vi "Test Write Enums.vi"(11 "TwinCAT ADS in":refnum<class "TwinCAT ADS.lvclass">) -> (3 "TwinCAT ADS out":refnum<class "TwinCAT ADS.lvclass">)   [LabVIEW 2018]
uses:
  TwinCAT ADS Class/TwinCAT ADS.lvclass
  Controls/Enum.ctl
  67abcce4-d906-4956-a77e-4a47c9dde040.vi
  c0c5b84e-43cd-4ba1-b01f-cca28dc7bea8.vi
  903064a7-6281-4536-8159-57f8726da337.vi
  a8d287bd-4485-4814-8cd1-9655769c98e5.vi
  TwinCAT ADS Class/VIs/Data/Read.vi
  <vilib>/addons/_JKI Toolkits/Caraya/classes/Assert/Assert Equal Value_Variant.vi
  <vilib>/addons/_JKI Toolkits/Caraya/classes/Test/Test.lvclass
  <vilib>/addons/_JKI Toolkits/Caraya/classes/Assert/Assert.lvclass
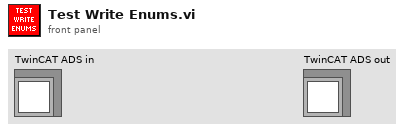
[diagram p1: front panel]
types:
  T1 = typedef "Enum.ctl" = enum16{"Member 0", "Member 1", "Member 2"}
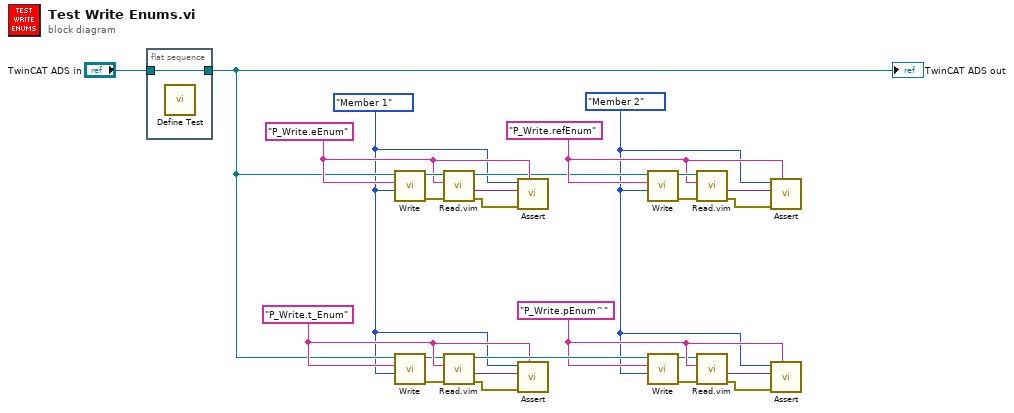
[diagram p0: block diagram]
diagram:
  w1 = Enum."Member 2" ("Enum")
  w2 = Enum."Member 1" ("Enum")
  w13 = "P_Write.pEnum^" ("Symbol Name")
  w8 = "P_Write.t_Enum" ("Symbol Name")
  w16 = "P_Write.refEnum" ("Symbol Name")
  w21 = "P_Write.eEnum" ("Symbol Name")
  n1 = flat-sequence {
    tunnel: "TwinCAT ADS in" -> [w27]
    tunnel: [w27] -> w3
    frame #0 {
      n2 = call <vilib>:"Define Test.vi"() -> ()  [unwired: 10 in, 2 out]
    }
  }
  n3 = call "Write.vi"("Value"=w2, "Symbol Name"=w21, "TwinCAT ADS in"=w3) -> ("error out"=w24:errorcluster, "TwinCAT ADS out"=w25:refnum<class "TwinCAT ADS.lvclass">)  [unwired: 7 in]
  n4 = call "Write.vi"("Value"=w2, "Symbol Name"=w8, "TwinCAT ADS in"=w3) -> ("error out"=w5:errorcluster, "TwinCAT ADS out"=w4:refnum<class "TwinCAT ADS.lvclass">)  [unwired: 7 in]
  n5 = call "Read.vim"("error in (no error)"=w24, "Symbol Name"=w21, "TwinCAT ADS in"=w25) -> ("error out"=w23:errorcluster, "Value"=w22:variant, "TwinCAT ADS out"=w15:refnum<class "TwinCAT ADS.lvclass">)  [unwired: 6 in]
  n6 = call "Read.vim"("error in (no error)"=w5, "Symbol Name"=w8, "TwinCAT ADS in"=w4) -> ("error out"=w6:errorcluster, "Value"=w7:variant, "TwinCAT ADS out"=w14:refnum<class "TwinCAT ADS.lvclass">)  [unwired: 6 in]
  n7 = call-poly <vilib>:"Assert.vi"("Label"=w21, "error in (no error)"=w23, "Y"=w22, "X"=w2) -> ()  [unwired: 6 in, 2 out]
  n8 = call-poly <vilib>:"Assert.vi"("Label"=w8, "error in (no error)"=w6, "Y"=w7, "X"=w2) -> ()  [unwired: 6 in, 2 out]
  n9 = call "Write.vi"("Value"=w1, "Symbol Name"=w16, "TwinCAT ADS in"=w15) -> ("error out"=w19:errorcluster, "TwinCAT ADS out"=w20:refnum<class "TwinCAT ADS.lvclass">)  [unwired: 7 in]
  n10 = call "Write.vi"("Value"=w1, "Symbol Name"=w13, "TwinCAT ADS in"=w14) -> ("error out"=w10:errorcluster, "TwinCAT ADS out"=w9:refnum<class "TwinCAT ADS.lvclass">)  [unwired: 7 in]
  n11 = call "Read.vim"("error in (no error)"=w19, "Symbol Name"=w16, "TwinCAT ADS in"=w20) -> ("error out"=w18:errorcluster, "Value"=w17:variant)  [unwired: 6 in, 1 out]
  n12 = call "Read.vim"("error in (no error)"=w10, "Symbol Name"=w13, "TwinCAT ADS in"=w9) -> ("error out"=w11:errorcluster, "Value"=w12:variant)  [unwired: 6 in, 1 out]
  n13 = call-poly <vilib>:"Assert.vi"("Label"=w16, "error in (no error)"=w18, "Y"=w17, "X"=w1) -> ()  [unwired: 6 in, 2 out]
  n14 = call-poly <vilib>:"Assert.vi"("Label"=w13, "error in (no error)"=w11, "Y"=w12, "X"=w1) -> ()  [unwired: 6 in, 2 out]
  "TwinCAT ADS out" <- w3
